vi "writeToXML.vi"(8 "error in (no error)":errorcluster, 10 "Class Label":string="Azimuth", 11 "Azimuth in":refnum<class "Azimuth.lvclass">) -> (0 "error out":errorcluster, 2 "XML out":string="<Azimuth>\n  <degreesArc>0</degreesArc>\n  <minutesArc>0</minutesArc>\n  <secondsArc>0</secondsArc>\n</Azimuth>", 3 "Azimuth out":refnum<class "Azimuth.lvclass">)   [LabVIEW 2014, in "TCSDataDefinitions.lvlib" / "TCSCommand.lvlib" / "TargetConfiguration.lvlib" / "Target.lvlib" / "FixedTarget.lvlib" / "Azimuth.lvclass"]
uses:
  Azimuth.lvclass
  <userlib>/Common/UnitsAndXML/FlattenItemWithUnitToXML/FlattenPlaneAngleToXML/PlaneAngleUnit.ctl
  Azimuth.lvclass/Azimuth.ctl
  <userlib>/Common/UnitsAndXML/UnitsAndXML.lvlib
  <userlib>/Common/XML/XMLGenerator/XMLGenerator.lvclass
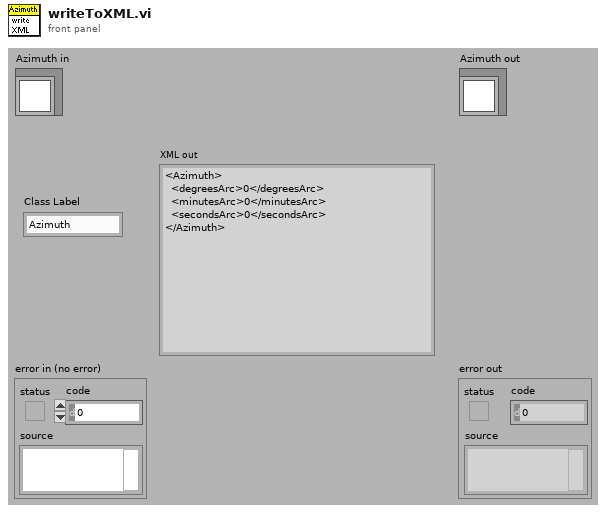
[diagram p1: front panel]
types:
  T1 = typedef "UnitsAndXML.lvlib/PlaneAngleUnit.ctl" = enum16{"rad", "deg", "'", "\""}
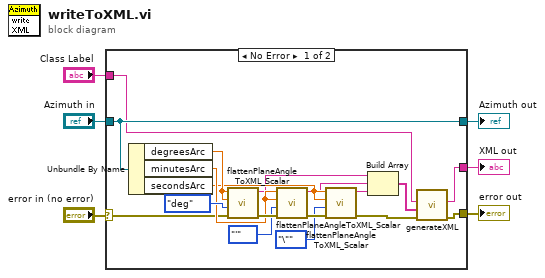
[diagram p0: block diagram]
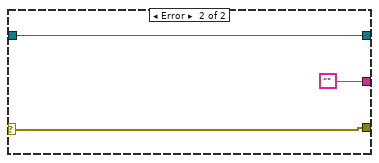
[diagram p2: hidden frame]
diagram:
  n1 = case shown="No Error" "error in (no error)" {
    selector: "error in (no error)" -> [w16 w27]
    tunnel: [w10 w27] -> w5
    tunnel: [w8 w26] -> w3
    tunnel: "Azimuth in" -> [w8 w26]
    tunnel: [w9 ""] -> w2
    tunnel: "Class Label" -> [w7 _]
    frame No Error {
      n2 = Unbundle By Name(w8) -> ("degreesArc"=w19:dbl[unit], "minutesArc"=w18:dbl[unit], "secondsArc"=w17:dbl[unit])
      n3 = call <userlib>:"flattenPlaneAngleToXML_Scalar.vi"("error in (no error)"=w16, "planeAngleUnitInXML"=PlaneAngleUnit."deg", "planeAngleAgain"=w19, "planeAngle"=w19) -> ("error out"=w22:errorcluster, "xmlString"=w14:string)  [unwired: 6 in]
      n4 = call <userlib>:"flattenPlaneAngleToXML_Scalar.vi"("error in (no error)"=w22, "planeAngleUnitInXML"=PlaneAngleUnit."'", "planeAngleAgain"=w18, "planeAngle"=w18) -> ("error out"=w24:errorcluster, "xmlString"=w13:string)  [unwired: 6 in]
      n5 = call <userlib>:"flattenPlaneAngleToXML_Scalar.vi"("error in (no error)"=w24, "planeAngleUnitInXML"=PlaneAngleUnit."\"", "planeAngleAgain"=w17, "planeAngle"=w17) -> ("error out"=w11:errorcluster, "xmlString"=w12:string)  [unwired: 6 in]
      n6 = Build Array(w14, w13, w12) -> (w15:string[])
      n7 = call <userlib>:"generateXML.vi"("error in"=w11, "childrenXML"=w15, "elementName"=w7) -> ("error out"=w10:errorcluster, "XML out"=w9:string)  [unwired: 6 in, 1 out]
    }
    frame Error {
    }
  }
  "error out" <- w5
  "Azimuth out" <- w3
  "XML out" <- w2
